vi "String to Str Hex Array.vi"(8 "error in (no error)":errorcluster, 10 "String":string, 11 "LED Matrix in":refnum<class "LED Matrix.lvclass">) -> (0 "error out":errorcluster, 1 "Right":string, 2 "Left":string, 3 "LED Matrix out":refnum<class "LED Matrix.lvclass">)   [LabVIEW 2026, in "LED Matrix.lvlib" / "LED Matrix.lvclass"]
uses:
  LED Matrix.lvclass
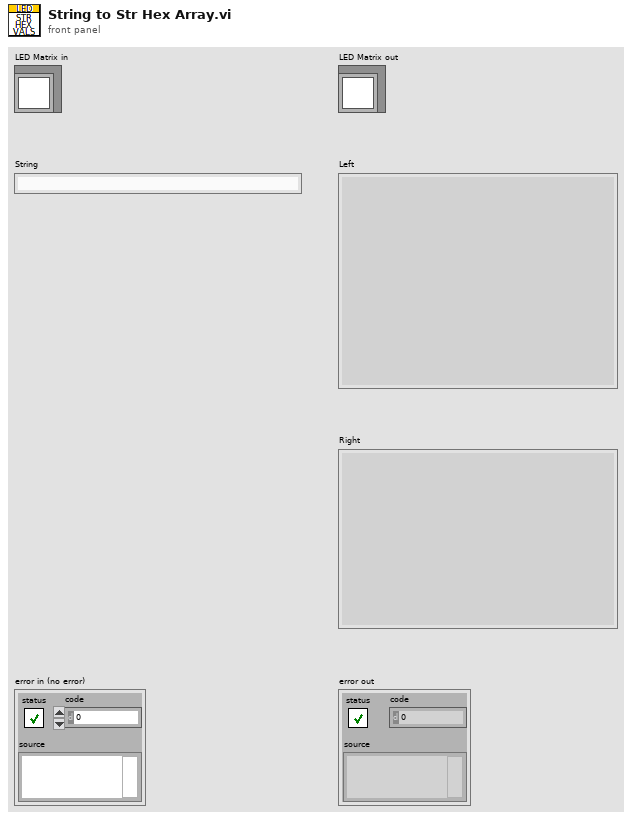
[diagram p1: front panel]
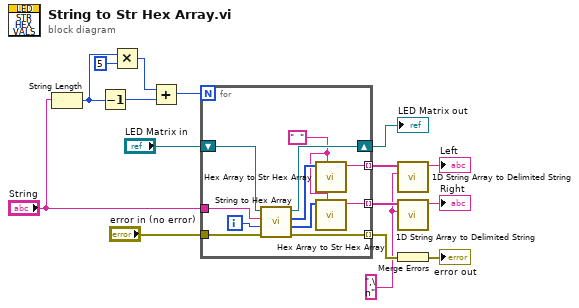
[diagram p0: block diagram]
diagram:
  w1 = ",\n" ("delimiter")
  n1 = String Length(string="String") -> (length=w7:i32)
  n2 = Decrement(x=w7) -> (x-1=w5:i32)
  n3 = Multiply(x=w7, y=5) -> (x*y=w6:i32)
  n4 = Add(x=w6, y=w5) -> (x+y=w4:i32)
  n5 = for {
    N: w4 -> [_]
    tunnel: "error in (no error)" -> [w27]
    tunnel: "String" -> [w24]
    shift-right: [w25] -> w14
    shift-left: "LED Matrix in" -> [w26]
    tunnel: [w22] -> w12 mode=indexing
    tunnel: [w20] -> w10 mode=indexing
    tunnel: [w18] -> w9 mode=indexing
    i -> [w23]
    w17 = "  " ("Pre-Line Pad")
    n6 = call "String to Hex Array.vi"("error in (no error)"=w27, "Offset"=w23, "String"=w24, "LED Matrix in"=w26) -> ("error out"=w22:errorcluster, "Right"=w19:u8[], "Left"=w21:u8[], "LED Matrix out"=w25:refnum<class "LED Matrix.lvclass">)  [unwired: 4 in]
    n7 = call "Hex Array to Str Hex Array.vi"("Pre-Line Pad"=w17, "Hex Array"=w21) -> ("Hex Value String"=w20:string)  [unwired: 9 in]
    n8 = call "Hex Array to Str Hex Array.vi"("Pre-Line Pad"=w17, "Hex Array"=w19) -> ("Hex Value String"=w18:string)  [unwired: 9 in]
  }
  "LED Matrix out" <- w14
  n9 = call <vilib>:"1D String Array to Delimited String.vi"("delimiter"=w1, "string array"=w10) -> ("delimited string"=→"Left":string)  [unwired: 9 in]
  n10 = call <vilib>:"1D String Array to Delimited String.vi"("delimiter"=w1, "string array"=w9) -> ("delimited string"=→"Right":string)  [unwired: 9 in]
  n11 = Merge Errors(w12) -> (→"error out":errorcluster)
